vi "Instrument Type ID.vi"() -> (1 "instrument type id":string="niDigitalPattern")   [LabVIEW 2020, in "MeasurementLink niDigital.lvlib" / "Session Factory.lvclass"]
uses:
  Session Factory.lvclass
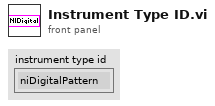
[diagram p1: front panel]
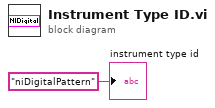
[diagram p0: block diagram]
diagram:
  "instrument type id" <- "niDigitalPattern" ("instrument type id")
